vi "Read_SubsystemName.vi"(8 "error in (no error)":errorcluster, 11 "SubsystemData in":refnum<class "SubsystemData.lvclass">) -> (0 "error out":errorcluster, 2 "Subsystem Name":string, 3 "SubsystemData out":refnum<class "SubsystemData.lvclass">)   [LabVIEW 2017, in "SubsystemData.lvclass"]
uses:
  SubsystemData.lvclass
  SubsystemData.lvclass/SubsystemData.ctl
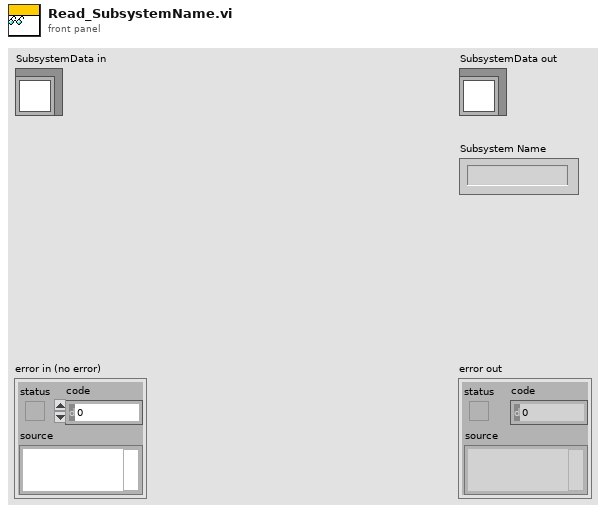
[diagram p1: front panel]
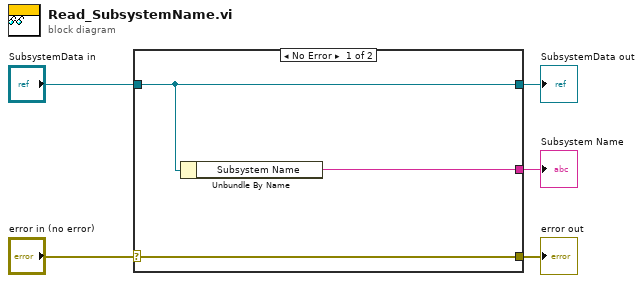
[diagram p0: block diagram]
diagram:
  n1 = case shown="No Error" "error in (no error)" {
    selector: "error in (no error)" -> [w8 w9]
    tunnel: [w8 w9] -> w4
    tunnel: [w7 w10] -> w2
    tunnel: "SubsystemData in" -> [w7 w10]
    tunnel: [w6 _] -> w1
    frame No Error {
      n2 = Unbundle By Name(w7) -> ("Subsystem Name"=w6:string)
    }
    frame Error {
    }
  }
  "error out" <- w4
  "SubsystemData out" <- w2
  "Subsystem Name" <- w1
